vi "bool_string.vi"(9 "boolean array":bool[](array[boolean]), 10 "FalseValue":string, 11 "TrueValue":string) -> (3 "string array":string[](array[string]))   [LabVIEW 2011]
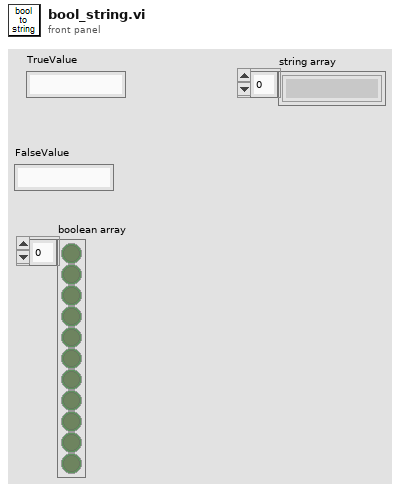
[diagram p1: front panel]
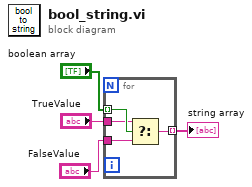
[diagram p0: block diagram]
diagram:
  n1 = for {
    tunnel: "boolean array" -> [w8] mode=indexing
    tunnel: "TrueValue" -> [w7]
    tunnel: "FalseValue" -> [w6]
    tunnel: [w5] -> w1 mode=indexing
    n2 = Select(t=w7, s=w8, f=w6) -> (s? t:f=w5:string)
  }
  "string array" <- w1
